vi "Read_Write_Trav_position.vi"(2 "Matched Configurations In":T1[](array[typedef]) {"Static Drive Configuration"."Indexer Mode  (FSA)" items=["Incremental", "Absolute"]; "Static Drive Configuration"."Buffer at Stop (SSH)" items=["Clear buffer", "Save and Continue"]; "Static Drive Configuration"."Buffer at Limit (SSG)" items=["Clear buffer", "Save and Continue"]; "Static Drive Configuration"."RS232 Echo Control (SSA)" items=["Echo ON", "Echo OFF"]; "Static Drive Configuration"."Reference edge of Home (OSH)" items=["CW", "CCW"]; "Static Drive Configuration"."Encoder Z for Home (OSD)" items=["Don't use", "Enable"]; "Static Drive Configuration"."Home Switch Sense (OSC)" items=["Normally Open", "Normally Closed"]; "Static Drive Configuration"."Home Position (OSB)" items=["Anywhere in Switch", "Edge of Switch"]; "Static Drive Configuration"."Limit Switch Sense (OSA)" items=["Normally Closed", "Normally Open"]; "Static Drive Configuration"."Limit Disable (LD)" items=["Both Enabled", "CW Disabled", "CCW Disabled", "Both Disabled"]; "Static Drive Configuration"."Stall Detect (FSH)" items=["Disable", "Enable"]; "Static Drive Configuration"."OP2 in Deadband (FSG)" items=["Don't Use", "ACTIVATE"]; "Static Drive Configuration"."Stop on Trigger 3 (FSF)" items=["Ignore", "STOP!"]; "Static Drive Configuration"."Activate OP1 on stall (FSE)" items=["Do not Activate", "ACTIVATE!"]; "Static Drive Configuration"."Stop on Stall (FSD)" items=["Continue", "STOP"]; "Static Drive Configuration"."Position Maintenance (FSC)" items=["Disabled", "Enabled"]; "Static Drive Configuration"."Step Mode  (FSB)" items=["Motor", "Encoder"]; "Static Drive Configuration"."Encoder Resolution (ER)" min=1 max=50000; "Static Drive Configuration"."Dead Band Window (DW)" min=0 max=999999999; "Static Drive Configuration"."Dead Band (DB)" min=0 max=999999999; "Static Drive Configuration"."Correction Gain % (CG)" items=["n/a", "12.5", "25", "37.5", "50", "62.5", "75", "87.5", "100"]; "Channel Properties"."Current Pos" format="%.2f"; "Channel Properties"."Backlash/Eng units" format="%.2f"; "Channel Properties"."Pulses/rev" format="%.2f"; "Channel Properties"."Pos Tolerance" format="%.2f"; "Channel Properties"."Pulses/unit" format="%.2f"; "Channel Properties"."Acc. Min" format="%.2f"; "Channel Properties"."Acc. Max" format="%.2f"; "Channel Properties"."Vel. Min" format="%.2f"; "Channel Properties"."Vel. Max" format="%.2f"; "Channel Properties"."Acc. Default" format="%.2f"; "Channel Properties"."Vel. Default" format="%.2f"}, 3 "Mode":T4(ring), 4 "Traverse Name":string="EnFlo Tunnel") -> (0 "Matched Configurations Out":T1[](array[typedef]) {"Static Drive Configuration"."Indexer Mode  (FSA)" items=["Incremental", "Absolute"]; "Static Drive Configuration"."Buffer at Stop (SSH)" items=["Clear buffer", "Save and Continue"]; "Static Drive Configuration"."Buffer at Limit (SSG)" items=["Clear buffer", "Save and Continue"]; "Static Drive Configuration"."RS232 Echo Control (SSA)" items=["Echo ON", "Echo OFF"]; "Static Drive Configuration"."Reference edge of Home (OSH)" items=["CW", "CCW"]; "Static Drive Configuration"."Encoder Z for Home (OSD)" items=["Don't use", "Enable"]; "Static Drive Configuration"."Home Switch Sense (OSC)" items=["Normally Open", "Normally Closed"]; "Static Drive Configuration"."Home Position (OSB)" items=["Anywhere in Switch", "Edge of Switch"]; "Static Drive Configuration"."Limit Switch Sense (OSA)" items=["Normally Closed", "Normally Open"]; "Static Drive Configuration"."Limit Disable (LD)" items=["Both Enabled", "CW Disabled", "CCW Disabled", "Both Disabled"]; "Static Drive Configuration"."Stall Detect (FSH)" items=["Disable", "Enable"]; "Static Drive Configuration"."OP2 in Deadband (FSG)" items=["Don't Use", "ACTIVATE"]; "Static Drive Configuration"."Stop on Trigger 3 (FSF)" items=["Ignore", "STOP!"]; "Static Drive Configuration"."Activate OP1 on stall (FSE)" items=["Do not Activate", "ACTIVATE!"]; "Static Drive Configuration"."Stop on Stall (FSD)" items=["Continue", "STOP"]; "Static Drive Configuration"."Position Maintenance (FSC)" items=["Disabled", "Enabled"]; "Static Drive Configuration"."Step Mode  (FSB)" items=["Motor", "Encoder"]; "Static Drive Configuration"."Encoder Resolution (ER)" min=1 max=50000; "Static Drive Configuration"."Dead Band Window (DW)" min=0 max=999999999; "Static Drive Configuration"."Dead Band (DB)" min=0 max=999999999; "Static Drive Configuration"."Correction Gain % (CG)" items=["n/a", "12.5", "25", "37.5", "50", "62.5", "75", "87.5", "100"]; "Channel Properties"."Current Pos" format="%.2f"; "Channel Properties"."Backlash/Eng units" format="%.2f"; "Channel Properties"."Pulses/rev" format="%.2f"; "Channel Properties"."Pos Tolerance" format="%.2f"; "Channel Properties"."Pulses/unit" format="%.2f"; "Channel Properties"."Acc. Min" format="%.2f"; "Channel Properties"."Acc. Max" format="%.2f"; "Channel Properties"."Vel. Min" format="%.2f"; "Channel Properties"."Vel. Max" format="%.2f"; "Channel Properties"."Acc. Default" format="%.2f"; "Channel Properties"."Vel. Default" format="%.2f"})   [LabVIEW 2011]
uses:
  AxisConfigCluster.ctl
  DriveProperties.ctl
  DriveStaticConfig.ctl
  Anemometry/Anemometry Sub Vis/Globals/Constants_global.vi
  DriveConfigGlobal.vi
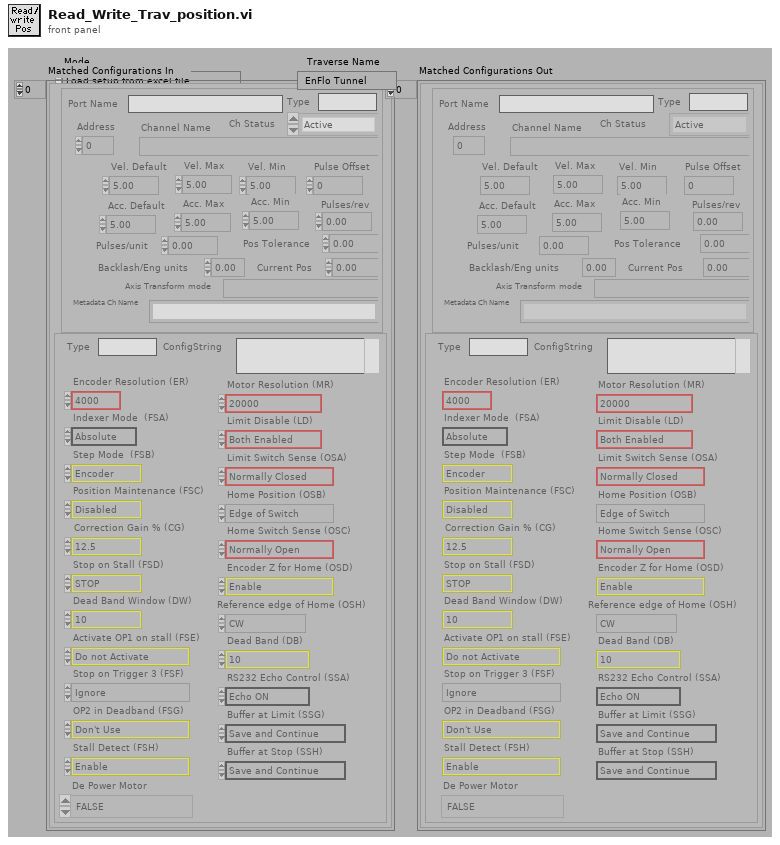
[diagram p1: front panel]
types:
  T1 = typedef "AxisConfigCluster.ctl" = cluster{"Channel Properties":T2, "Static Drive Configuration":T3}
  T2 = typedef "DriveProperties.ctl" = cluster{"Channel Name":string, "Vel. Default":dbl, "Acc. Default":dbl, "Vel. Max":dbl, "Vel. Min":dbl, "Acc. Max":dbl, "Acc. Min":dbl, "Pulses/unit":dbl, "Address":u8, "Pulse Offset":i32, "Pos Tolerance":dbl, "Pulses/rev":dbl, "Backlash/Eng units":dbl, "Current Pos":dbl, "Ch Status":enum16{"Active", "Offline", "Simulate"}, "Port Name":string, "Axis Transform mode":string, "Metadata Ch Name":string, "Type":string}
  T3 = typedef "DriveStaticConfig.ctl" = cluster{"Correction Gain % (CG)":u16, "Dead Band (DB)":i32, "Dead Band Window (DW)":i32, "Encoder Resolution (ER)":i32, "Step Mode  (FSB)":u16, "Position Maintenance (FSC)":u16, "Stop on Stall (FSD)":u16, "Activate OP1 on stall (FSE)":u16, "Stop on Trigger 3 (FSF)":u16, "OP2 in Deadband (FSG)":u16, "Stall Detect (FSH)":u16, "Limit Disable (LD)":u16, "Motor Resolution (MR)":enum16{"200", "400", "1000", "2000", "4000", "5000", "10000", "12800", "18000", "20000", "21600", "25000", "25400", "25600", "36000", "50000", "278528", "425984", "507904", "614400", "655360", "819200", "1024000"}, "Limit Switch Sense (OSA)":u16, "Home Position (OSB)":u16, "Home Switch Sense (OSC)":u16, "Encoder Z for Home (OSD)":u16, "Reference edge of Home (OSH)":u16, "RS232 Echo Control (SSA)":u16, "Buffer at Limit (SSG)":u16, "Buffer at Stop (SSH)":u16, "Indexer Mode  (FSA)":u16, "Type":string, "ConfigString":string, "De Power Motor":enum16{"TRUE", "FALSE"}}
  T4 = enum16{"Load setup from excel file", "Save setup to excel file"}
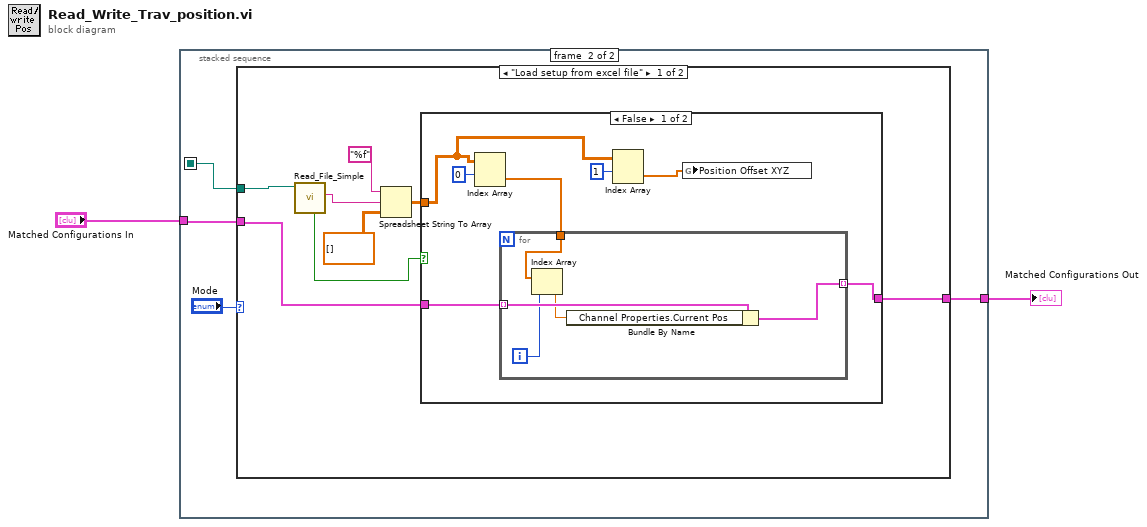
[diagram p0: block diagram]
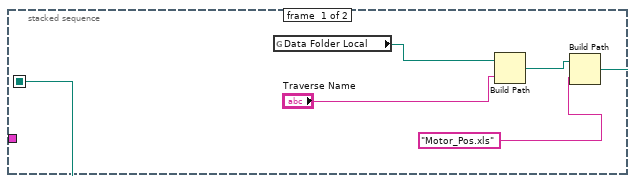
[diagram p2: hidden frame]
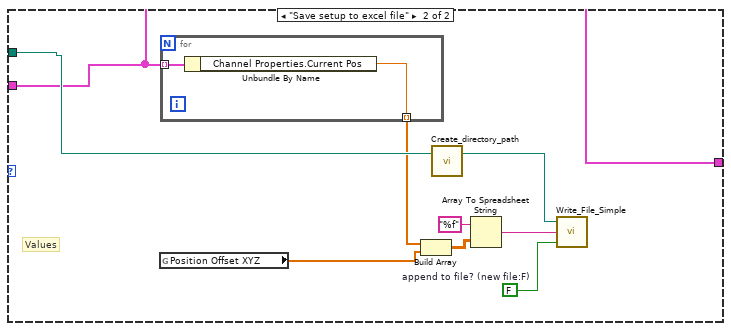
[diagram p4: hidden frame]
diagram:
  n1 = stacked-sequence {
    seq-local: [w4 _] -> [_ w10]
    tunnel: "Matched Configurations In" -> [_ w9]
    tunnel: [_ w8] -> w1
    frame #0 {
      n2 = global read "Constants_global.vi" "Data Folder Local"() -> (w5:path)
      n3 = Build Path(base path=w5, name or relative path="Traverse Name") -> (appended path=w3:path)
      n4 = Build Path(base path=w3, name or relative path="Motor_Pos.xls" ("Substring")) -> (appended path=w4:path)
    }
    frame #1 {
      n5 = case shown="\"Load setup from excel file\"" "Mode" {
        tunnel: w10 -> [w19 w37]
        tunnel: w9 -> [w18 w36]
        tunnel: [w17 w36] -> w8
        frame "Load setup from excel file" {
          n6 = call "Read_File_Simple.vi"("Filename"=w19) -> ("Error?"=w13:bool, "string"=w14:string)  [unwired: 2 in, 6 out]
          n7 = Spreadsheet String To Array(format string="%f", spreadsheet string=w14, array type (2D Dbl)=dbl[][] []) -> (array=w12:dbl[][])  [unwired: 1 out]
          n8 = case shown="False" w13 {
            tunnel: w18 -> [w26 w32]
            tunnel: [w25 w32] -> w17
            tunnel: w12 -> [w21 _]
            frame False {
              n9 = Index Array(array=w21, index (row)=0) -> (element=w23:dbl[])  [unwired: 1 in]
              n10 = for {
                tunnel: w26 -> [w31] mode=indexing
                tunnel: [w30] -> w25 mode=indexing
                tunnel: w23 -> [w29]
                i -> [w28]
                n11 = Index Array(array=w29, index=w28) -> (element=w27:dbl)
                n12 = Bundle By Name(cluster=w31, "Channel Properties.Current Pos"=w27) -> (w30:T1)
              }
              n13 = Index Array(array=w21, index (row)=1) -> (element=w20:dbl[])  [unwired: 1 in]
              n14 = global write "DriveConfigGlobal.vi" "Position Offset XYZ"(w20) -> ()
            }
            frame True {
            }
          }
        }
        frame "Save setup to excel file" {
          w39 = FALSE  # append to file? (new file:F)
          # "Values"
          n15 = global read "DriveConfigGlobal.vi" "Position Offset XYZ"() -> (w34:dbl[])
          n16 = for {
            tunnel: w36 -> [w43] mode=indexing
            tunnel: [w42] -> w35 mode=indexing
            n17 = Unbundle By Name(w43) -> ("Channel Properties.Current Pos"=w42:dbl)
          }
          n18 = Build Array(w35, w34) -> (w33:dbl[][])
          n19 = call "Create_directory_path.vi"("Path name"=w37) -> ("Path name Out"=w41:path)  [unwired: 1 in, 1 out]
          n20 = Array To Spreadsheet String(array=w33, 3:"%f" ("format string")) -> (spreadsheet string=w40:string)  [unwired: 1 out]
          n21 = call "Write_File_Simple.vi"("append to file? (new file:F)"=w39, "character string"=w40, "file path"=w41) -> ()  [unwired: 2 out]
        }
      }
    }
  }
  "Matched Configurations Out" <- w1
